vi "Communication - Ping.vi"(8 "error in":errorcluster, 11 "IP":string) -> (0 "error out":errorcluster, 2 "standard output":string, 3 "Active?":bool)   [LabVIEW 2019]
uses:
  <vilib>/Utility/file.llb/Read Delimited Spreadsheet (string).vi
panel:
  out "all rows":string[][](array[string])
  out "index":i32
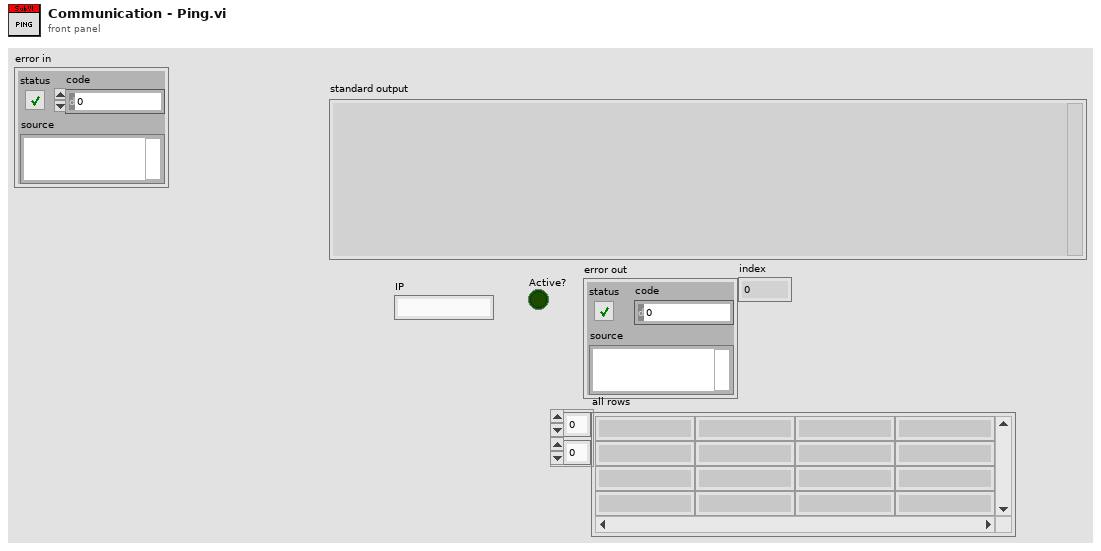
[diagram p1: front panel]
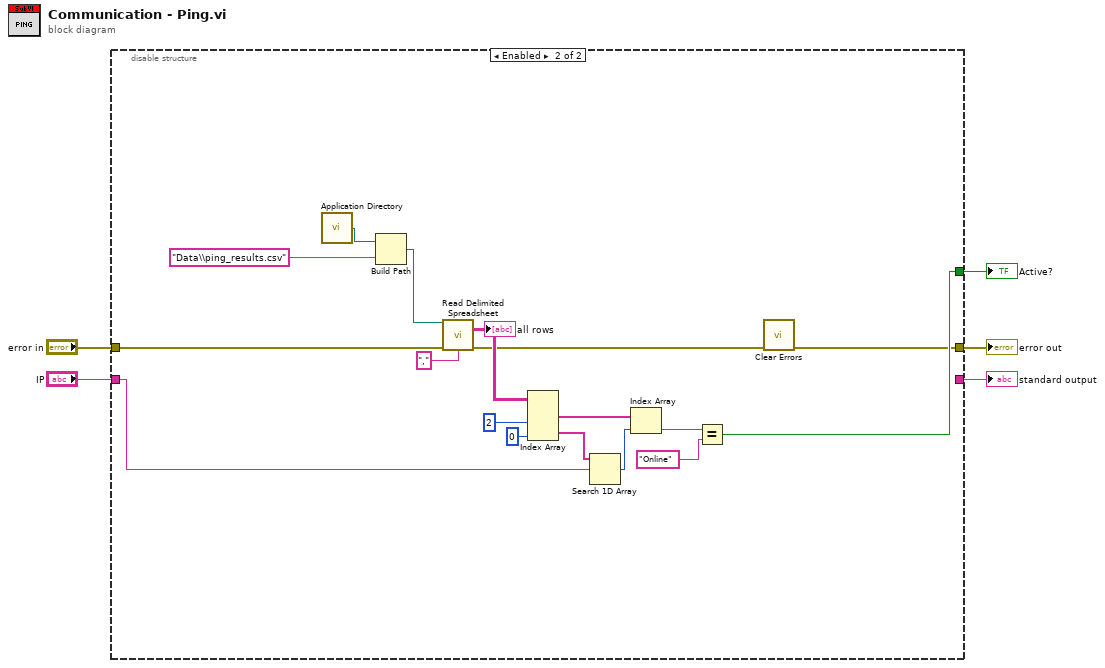
[diagram p0: block diagram]
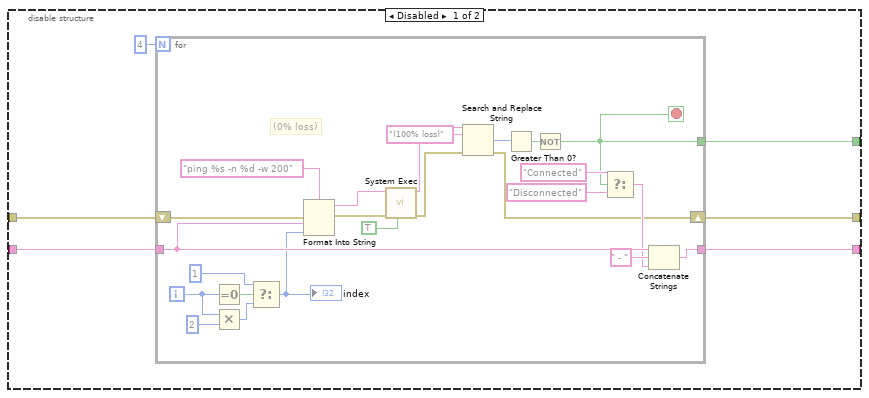
[diagram p2: hidden frame]
diagram:
  n1 = disable-structure shown="Enabled" {
    disable-tunnel: "IP" -> [w11 w45]
    disable-tunnel: [w10 _] -> w4
    disable-tunnel: [w9 w38] -> w3
    disable-tunnel: "error in" -> [w8 w49]
    disable-tunnel: [w7 w36] -> w1
    frame Disabled {
      n2 = for {
        N: 4 -> [_]
        tunnel: [w12] -> w9
        shift-right: [w20] -> w7
        shift-left: w8 -> [w21]
        tunnel: w11 -> [w28]
        tunnel: [w27] -> w10
        i -> [w16]
        stop <- w12 stop-if-true
        # "(0% loss)"
        n3 = Equal To 0?(x=w16) -> (x = 0?=w18:bool)
        n4 = Multiply(x=w16, y=2) -> (x*y=w14:i32)
        n5 = Select(t=1, s=w18, f=w14) -> (s? t:f=w13:i32)
        "index" <- w13
        n6 = Format Into String(format string="ping %s -n %d -w 200" ("command line"), error in=w21, w28, w13) -> (resulting string=w19:string, error out=w32:errorcluster)  [unwired: 1 in]
        n7 = call <vilib>:"System Exec.vi"("run minimized? (F)"=TRUE, "error in (no error)"=w32, "command line"=w19) -> ("error out"=w30:errorcluster, "standard output"=w25:string)  [unwired: 5 in, 2 out]
        n8 = Search and Replace String(input string=w25, search string="(100% loss)", error in=w30) -> (number of replacements=w29:i32, error out=w20:errorcluster)  [unwired: 5 in, 2 out]
        n9 = Greater Than 0?(x=w29) -> (x > 0?=w33:bool)
        n10 = Not(x=w33) -> (.not. x?=w12:bool)
        n11 = Select(t="Connected" ("search string"), s=w12, f="Disconnected" ("search string")) -> (s? t:f=w23:string)
        n12 = Concatenate Strings(w28, " - " ("string"), w23) -> (w27:string)
      }
    }
    frame Enabled {
      n13 = call <vilib>:"Application Directory.vi"() -> ("Application Directory"=w52:path)
      n14 = Build Path(base path=w52, name or relative path="Data\\ping_results.csv") -> (appended path=w50:path)
      n15 = call-poly <vilib>:"Read Delimited Spreadsheet.vi"("file path (dialog if empty)"=w50, "error in (no error)"=w49, "delimiter (\\t)"="," ("delimiter (\\t)")) -> ("all rows"=w48:string[][], "error out"=w37:errorcluster)  [unwired: 7 in, 4 out]
      "all rows" <- w48
      n16 = Index Array(array=w48, index (col) #1=2 ("disabled index (col)"), index (col) #2=0 ("disabled index (col)")) -> (element #1=w43:string[], element #2=w46:string[])  [unwired: 2 in]
      n17 = Search 1D Array(1D array=w46, element=w45) -> (index of element=w42:i32)  [unwired: 1 in]
      n18 = Index Array(array=w43, index=w42) -> (element=w40:string)
      n19 = Equal?(x=w40, y="Online") -> (x = y?=w38:bool)
      n20 = call <vilib>:"Clear Errors.vi"("error in (no error)"=w37) -> ("error out"=w36:errorcluster)  [unwired: 5 in, 1 out]
    }
  }
  "Active?" <- w3
  "standard output" <- w4
  "error out" <- w1
